vi "ConfigMeasurement.vi"(8 "error in (no error)":errorcluster, 11 "NISTSamplerPluginsBase in":refnum<class "SamplerPluginsBase.lvclass">) -> (0 "error out":errorcluster, 3 "NISTSamplerPluginsBase out":refnum<class "SamplerPluginsBase.lvclass">)   [LabVIEW 2014, in "SamplerPlugins.lvlib" / "SamplerPluginsBase.lvclass"]
uses:
  SamplerPluginsBase.lvclass
  <userlib>/NIST/BaseClasses/Object_class/BaseObject.lvclass
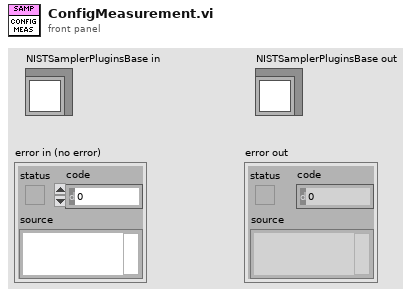
[diagram p1: front panel]
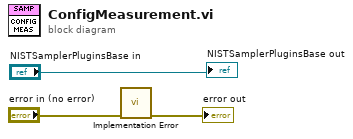
[diagram p0: block diagram]
diagram:
  n1 = call <userlib>:"Implementation Error.vi"("error in (no error)"="error in (no error)") -> ("error out"=→"error out":errorcluster)  [unwired: 10 in]
  "NISTSamplerPluginsBase out" <- "NISTSamplerPluginsBase in"
